vi "SensorDAQTest.vi"() -> ()   [LabVIEW 2018]
uses:
  87fd6717-2e3d-40a7-96cd-4556beea845e.vi
panel:
  in  "SetState":T1(ring)
  out "SensorReadings":dbl[](array[numeric])
  out "Sensor State":string
  # "Load Cell DAQ Unit Test Procedure:\n\nReturn the system to the default state after each test.\n\nTest Setup:\nPower on and connect to the DAQ Box\nAttach load cell the the appropriate plug on the DAQ box, place on the ground\nSet aside a set of weights and prepare means to balance them on the load cell\n\n1) Place weights on the load cell\n        Verify that each weight detected is accurate to 2%\n        Verify that no log has been created at C:/LPLDocs\n2) Set State to Record and run test 1\n        Verify that Sensor State matches Set State at all times\n        Verify that a log file has been created in C:/LPLDocs\n        Verify that the readings contained in the log are accurate and include accurate time data in the X column\n        Verify that the data rate in the log file is <= 50Hz\n3) Set State to Record, then to Overdrive\n        Verify that Sensor State matches Set State at all times\n        Verify that the data rate in the log file starts at <=50Hz, then jumps up to >1600 Hz\n4) Set State to Record, then to Pause\n        Verify that Sensor State matches Set State at all times\n        Verify that Sensor Readings freezes once the state is Pause\n        Verify that the log file contains data which ends at the point where the state is Pause"
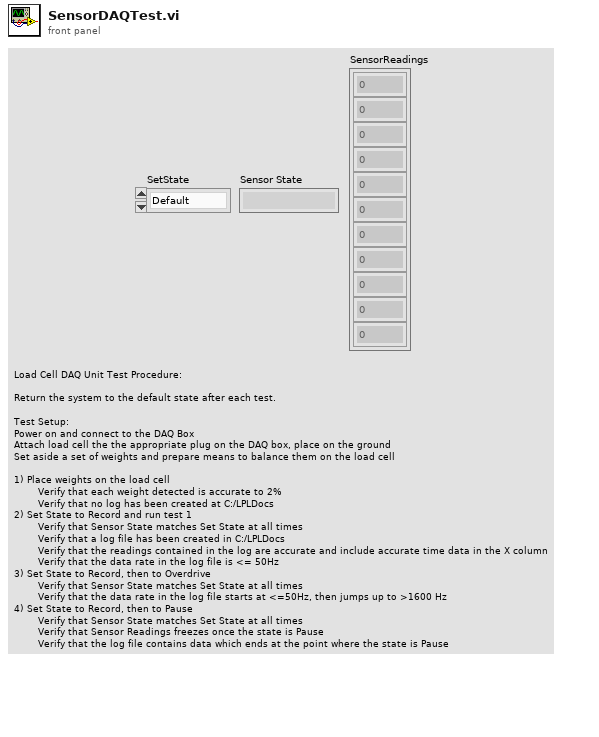
[diagram p1: front panel]
types:
  T1 = enum16{"Default", "Record", "Overdrive", "Pause"}
  T2 = cluster{"Sensors":refnum<notifier>, "LoadCell":refnum<notifier>, "FileOut":refnum<notifier>, "UI":refnum<notifier>}
  T3 = enum16{"Normal", "Overdrive", "Ready for Overdrive End", "Ready for new file", "New file"}
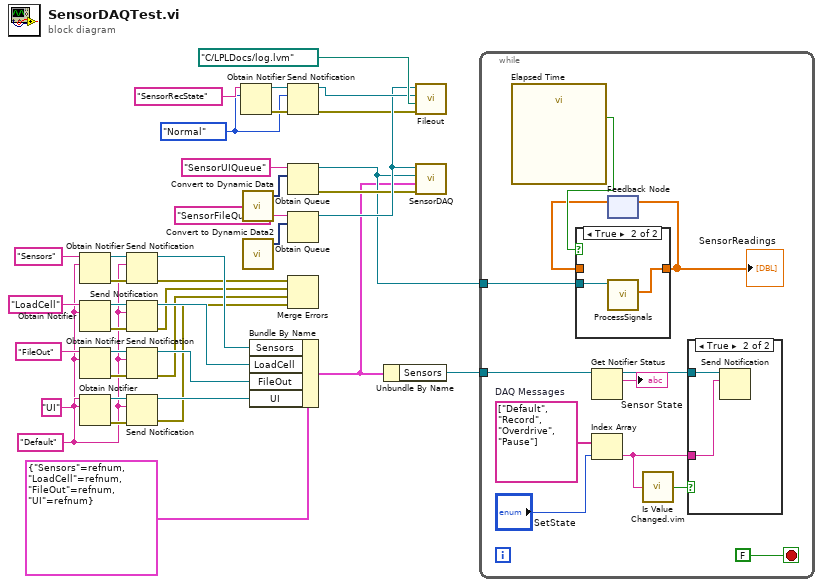
[diagram p0: block diagram]
diagram:
  w18 = "Default" ("RecState")
  w35 = T3."Normal" ("RecState")
  n1 = Obtain Notifier(name (unnamed)="Sensors", notification data type=w18) -> (notifier out=w20:refnum<notifier>, error out=w19:errorcluster)  [unwired: 2 in, 1 out]
  n2 = Obtain Notifier(name (unnamed)="LoadCell", notification data type=w18) -> (notifier out=w22:refnum<notifier>, error out=w23:errorcluster)  [unwired: 2 in, 1 out]
  n3 = Obtain Notifier(name (unnamed)="FileOut", notification data type=w18) -> (notifier out=w24:refnum<notifier>, error out=w25:errorcluster)  [unwired: 2 in, 1 out]
  n4 = Obtain Notifier(name (unnamed)="UI", notification data type=w18) -> (notifier out=w26:refnum<notifier>, error out=w27:errorcluster)  [unwired: 2 in, 1 out]
  n5 = Send Notification(notification=w18, notifier=w20, error in (no error)=w19) -> (notifier out=w15:refnum<notifier>, error out=w11:errorcluster)
  n6 = Send Notification(notification=w18, notifier=w22, error in (no error)=w23) -> (notifier out=w14:refnum<notifier>, error out=w10:errorcluster)
  n7 = Send Notification(notification=w18, notifier=w24, error in (no error)=w25) -> (notifier out=w13:refnum<notifier>, error out=w9:errorcluster)
  n8 = Send Notification(notification=w18, notifier=w26, error in (no error)=w27) -> (notifier out=w16:refnum<notifier>, error out=w12:errorcluster)
  n9 = Obtain Notifier(name (unnamed)="SensorRecState", notification data type=w35) -> (notifier out=w36:refnum<notifier>, error out=w37:errorcluster)  [unwired: 2 in, 1 out]
  n10 = call "Convert to Dynamic Data"() -> ("Dynamic Data Type"=w33:dynamicdata)  [unwired: 4 in]
  n11 = call "Convert to Dynamic Data2"() -> ("Dynamic Data Type"=w31:dynamicdata)  [unwired: 4 in]
  n12 = Bundle By Name(cluster=T2 {"Sensors"=refnum, "LoadCell"=refnum, "FileOut"=refnum, "UI"=refnum} ("Message Notifiers"), "Sensors"=w15, "LoadCell"=w14, "FileOut"=w13, "UI"=w16) -> (w2:T2)
  n13 = Send Notification(notification=w35, notifier=w36, error in (no error)=w37) -> (notifier out=w7:refnum<notifier>, error out=w5:errorcluster)
  n14 = Obtain Queue(name (unnamed)="SensorUIQueue", element data type=w33) -> (queue out=w3:refnum<queue>, error out=w4:errorcluster)  [unwired: 3 in, 1 out]
  n15 = Obtain Queue(name (unnamed)="SensorFileQueue", element data type=w31) -> (queue out=w6:refnum<queue>)  [unwired: 3 in, 2 out]
  n16 = Merge Errors(w11, w10, w9, w12) -> ()  [unwired: 1 out]
  n17 = Unbundle By Name(w2) -> ("Sensors"=w1:refnum<notifier>)
  n18 = call "Fileout.vi"("error in (no error)"=w5, "Filepath"=path "C:/LPLDocs/log.lvm", "RecState"=w7, "Logging Queue"=w6) -> ()  [unwired: 7 in, 1 out]
  n19 = call "SensorDAQ.vi"("error in (no error)"=w4, "Message Notifiers"=w2, "UI Queue"=w3, "Logging Queue"=w6) -> ()  [unwired: 7 in, 1 out]
  n20 = while {
    tunnel: w3 -> [w43]
    tunnel: w1 -> [w46]
    stop <- FALSE stop-if-true
    w50 = string[] ["Default", "Record", "Overdrive", "Pause"]  # DAQ Messages
    n21 = call "Elapsed Time"() -> ("Time has Elapsed"=w42:bool)  [unwired: 12 in, 7 out]
    n22 = Get Notifier Status(notifier=w46) -> (notifier out=w45:refnum<notifier>, current notification=→"Sensor State":string)  [unwired: 1 in, 3 out]
    n23 = Index Array(array=w50, index="SetState") -> (element=w47:string)
    n24 = feedback #1() -> (w40:dbl[])  [unwired: 1 in]
    n25 = case shown="True" w42 {
      tunnel: w43 -> [_ w53]
      tunnel: [w51 w52] -> w41
      tunnel: w40 -> [w51 _]
      frame False {
      }
      frame True {
        n26 = call "ProcessSignals.vi"("UI Queue"=w53) -> ("Array"=w52:dbl[])  [unwired: 9 in, 1 out]
      }
    }
    "SensorReadings" <- w41
    n27 = feedback-in #1(w41) -> ()
    n28 = call "Is Value Changed.vim"("value"=w47) -> ("changed or first call?"=w48:bool)
    n29 = case shown="True" w48 {
      tunnel: w47 -> [_ w55]
      tunnel: w45 -> [_ w54]
      frame False {
      }
      frame True {
        n30 = Send Notification(notification=w55, notifier=w54) -> ()  [unwired: 1 in, 2 out]
      }
    }
  }
